vi "6 Drive Set.vi"(0 "Motor devRevs":T1, 1 "Left side speed":dbl, 2 "Right side speed":dbl, 3 "error in (no error)":errorcluster) -> (7 "Motor devRevs":T1, 10 "error out":errorcluster)   [LabVIEW 2013]
uses:
  Drive Motors Typedef.ctl
  GearBox Typedef.ctl
  <vilib>/Rock Robotics/WPI/MotorControl/WPI_MotorControlDeviceRef.ctl
  <vilib>/Rock Robotics/SystemInterfaces/Typedef/FPGA_TypedefDigitalModule.ctl
  <vilib>/Rock Robotics/SystemInterfaces/DIO/FPGA_DIOPWMChannel.ctl
  <vilib>/Rock Robotics/WPI/PWM/WPI_PWMDeadband.ctl
  <vilib>/Rock Robotics/WPI/CAN/Jaguar/SubVIs/WPI_CANJaguar_ControlMode.ctl
  <vilib>/Rock Robotics/WPI/PWM/WPI_PWMTransform_ConPane.ctl
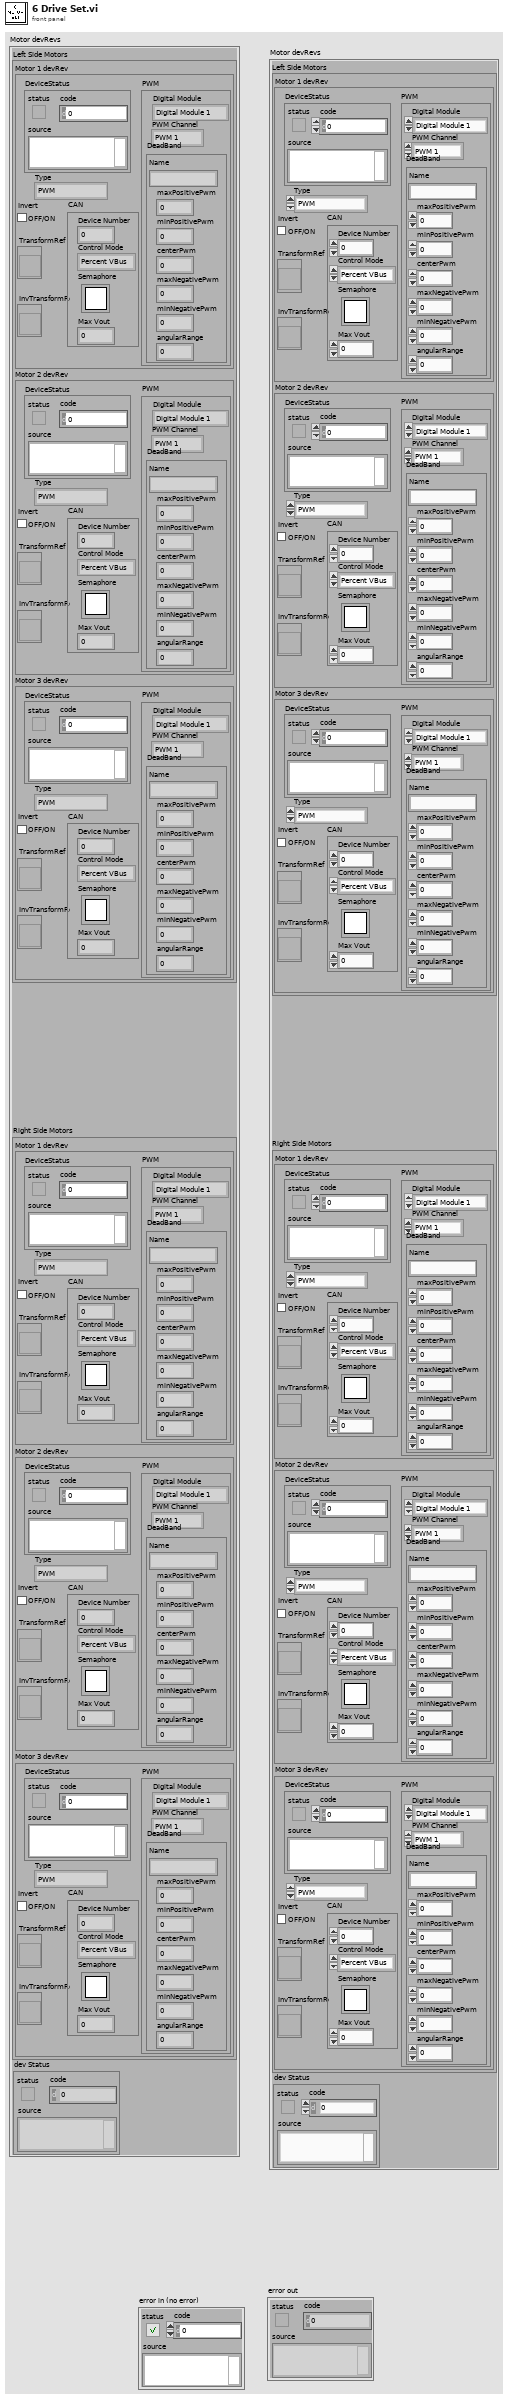
[diagram p1: front panel]
types:
  T1 = typedef "Drive Motors Typedef.ctl" = cluster{"Left Side Motors":T2, "Right Side Motors":T2, "dev Status":errorcluster}
  T2 = typedef "GearBox Typedef.ctl" = cluster{"Motor 1 devRev":T3, "Motor 2 devRev":T3, "Motor 3 devRev":T3}
  T3 = typedef "WPI_MotorControlDeviceRef.ctl" = cluster{"DeviceStatus":errorcluster, "Type":enum16{"PWM", "CAN"}, "PWM":cluster{"Digital Module":T4, "PWM Channel":T5, "DeadBand":T6}, "CAN":cluster{"Device Number":u8, "Control Mode":T7, "Semaphore":T8, "Max Vout":dbl}, "Invert":bool, "TransformRef":T9, "InvTransformRef":T9}
  T4 = typedef "FPGA_TypedefDigitalModule.ctl" = enum16{"Digital Module 1", "Digital Module 2"}
  T5 = typedef "FPGA_DIOPWMChannel.ctl" = enum8{"PWM 1", "PWM 2", "PWM 3", "PWM 4", "PWM 5", "PWM 6", "PWM 7", "PWM 8", "PWM 9", "PWM 10", "Invalid"}
  T6 = typedef "WPI_PWMDeadband.ctl" = cluster{"Name":string, "maxPositivePwm":i32, "minPositivePwm":i32, "centerPwm":i32, "maxNegativePwm":i32, "minNegativePwm":i32, "angularRange":u16}
  T7 = typedef "WPI_CANJaguar_ControlMode.ctl" = enum8{"Percent VBus", "Current", "Speed", "Position", "Voltage"}
  T8 = typedef "Semaphore RefNum" = refnum<k1>
  T9 = typedef "WPI_PWMTransform_ConPane.ctl" = refnum<vi>
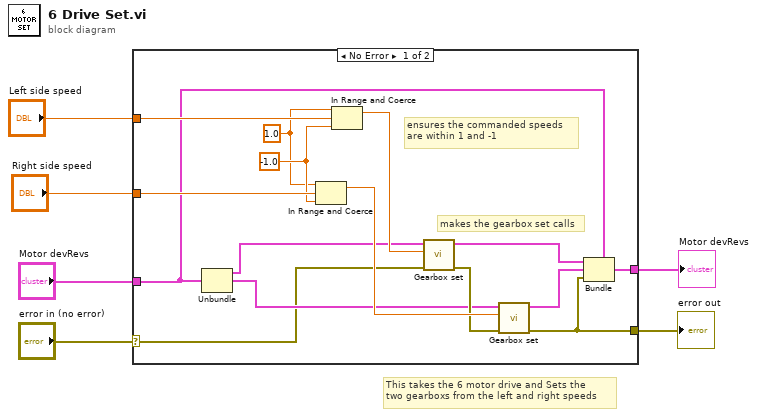
[diagram p0: block diagram]
diagram:
  # "This takes the 6 motor drive and Sets the\ntwo gearboxs from the left and right speeds"
  n1 = case shown="No Error" "error in (no error)" {
    selector: "error in (no error)" -> [w8 w22]
    tunnel: "Left side speed" -> [w21 _]
    tunnel: "Right side speed" -> [w20 _]
    tunnel: [w19 w23] -> w1
    tunnel: [w7 w22] -> w4
    tunnel: "Motor devRevs" -> [w18 w23]
    frame No Error {
      w16 = -1.0 ("lower limit")
      w15 = 1.0 ("upper limit")
      # "makes the gearbox set calls"
      # "ensures the commanded speeds\nare within 1 and -1"
      n2 = Unbundle(w18) -> ("Left Side Motors"=w9:T2, "Right Side Motors"=w10:T2)  [unwired: 1 out]
      n3 = In Range and Coerce(upper limit=w15, x=w20, lower limit=w16) -> (coerced(x)=w17:dbl)  [unwired: 1 out]
      n4 = In Range and Coerce(upper limit=w15, x=w21, lower limit=w16) -> (coerced(x)=w14:dbl)  [unwired: 1 out]
      n5 = call "Gearbox set.vi"("error in"=w8, "Gearbox Speed"=w14, "Gearbox Motors"=w9) -> ("error out"=w11:errorcluster, "Gearbox Motors dev rev"=w12:T2)  [unwired: 7 in]
      n6 = call "Gearbox set.vi"("error in"=w11, "Gearbox Speed"=w17, "Gearbox Motors"=w10) -> ("error out"=w7:errorcluster, "Gearbox Motors dev rev"=w13:T2)  [unwired: 7 in]
      n7 = Bundle(cluster=w18, "Left Side Motors"=w12, "Right Side Motors"=w13, "dev Status"=w7) -> (w19:T1)
    }
    frame Error {
      # "ERROR don't do anything"
    }
  }
  "error out" <- w4
  "Motor devRevs" <- w1
